vi "Display Telemtery Data.vi"(0 "Instance Details":T1) -> (17 "TX Queue State":i32(slide) scale=0.0..50.0, 18 "Initialisation Progress":u8(slide) scale=0.0..100.0, 19 "RX Queue State":i32(slide) scale=0.0..50.0, 20 "Drone Information Out":T4={"Heart Beat"=FALSE, "Aircraft ID"=0, "Tag ID"="", "System Status"="", "Base Mode"={"Custom Mode"=FALSE, "Test Enabled"=FALSE, "Autonomous Mode"=FALSE, "Guided Mode"=FALSE, "Stabilization Enabled"=FALSE, "HIL Enabled"=FALSE, "Manual Mode"=FALSE, "Arm"=FALSE}, "Armed/Disarmed"=FALSE, "Battery Voltage"=0.0, "Control Mode"=enum."Stabalise", "Initialisation"=0, "Heart Beat Status"=FALSE, "Mode"="", "Mission Uploaded"=FALSE} {"Initialisation" scale=0.0..100.0}, 21 "System Status Out":T9 {"Communication Drop Rate (%)" scale=0.0..100.0; "Battery Remaining (%)" scale=0.0..100.0; "CPU Load (%)" scale=0.0..100.0}, 22 "Status text":string, 23 "Armed/Disarmed":bool, 24 "Aircraft RC Data Out":T8, 25 "Aircraft Att Data Out":T7, 26 "Control Mode":T6=enum."Stabalise")   [LabVIEW 2014]
uses:
  Aircraft Information/Controls/Aircraft Sensor Status Data.ctl
  GUI Design/Indicators/Sensor Status LED CLuster.ctl
  GUI Design/Indicators/Status LED.ctl
  Aircraft Information/Controls/Aircraft Mode.ctl
  Aircraft Information/Controls/Aircraft RC Data.ctl
  Aircraft Information/Controls/Aircraft Attitude Data.ctl
  Aircraft Information/Controls/Drone Information.ctl
  Aircraft Information/Controls/Base Mode.ctl
  Ground Station to Aircraft Coms/SubVI/Aircraft Data Router/Controls/Known Aircraft.ctl
  Ground Station to Aircraft Coms/SubVI/Hardware Driver/Controls/Coms Driver Interface.ctl
  Controls/Telemetry Connection Type.ctl
  Aircraft Information/Sub VI/Get Aircraft Attitude.vi
  Aircraft Information/Sub VI/Get Aircraft RC.vi
  Aircraft Information/Sub VI/Get Aircraft System Status.vi
  Aircraft Information/Sub VI/Get Aircraft Information.vi
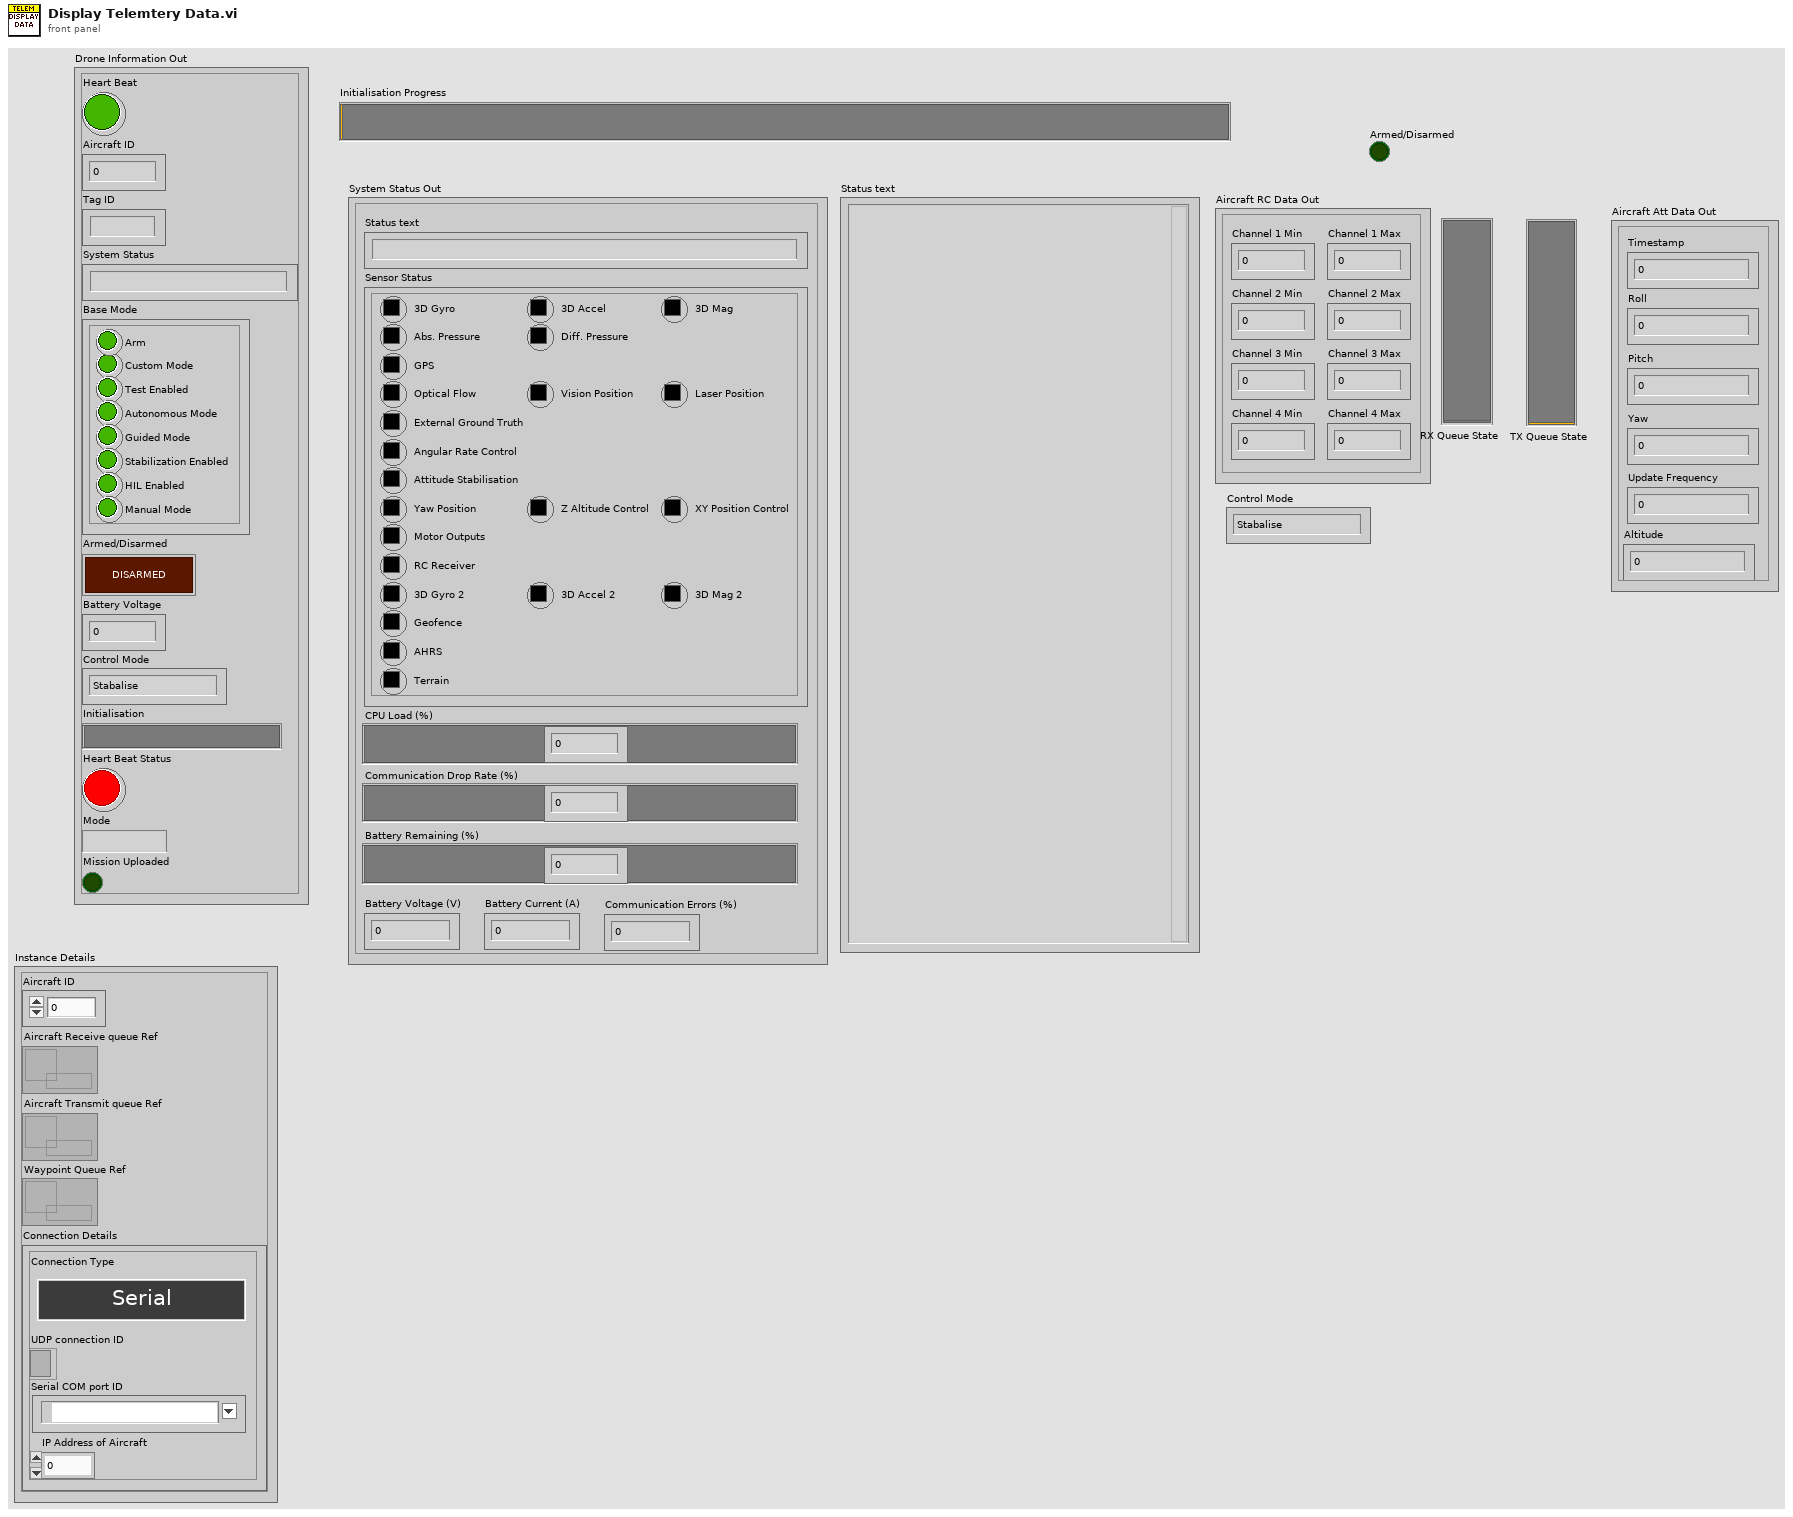
[diagram p1: front panel]
types:
  T1 = typedef "Known Aircraft.ctl" = cluster{"Aircraft ID":u8, "Aircraft Receive queue Ref":refnum<queue>, "Aircraft Transmit queue Ref":refnum<queue>, "Waypoint Queue Ref":refnum<queue>, "Connection Details":T2}
  T2 = typedef "Coms Driver Interface.ctl" = cluster{"Connection Type":T3, "UDP connection ID":refnum<k16>, "Serial COM port ID":refnum<visa-resource-name>, "IP Address of Aircraft":u32}
  T3 = typedef "Telemetry Connection Type.ctl" = enum16{"Serial", "UDP", "TCP"}
  T4 = typedef "Drone Information.ctl" = cluster{"Heart Beat":bool, "Aircraft ID":u8, "Tag ID":string, "System Status":string, "Base Mode":T5, "Armed/Disarmed":bool, "Battery Voltage":dbl, "Control Mode":T6, "Initialisation":u8, "Heart Beat Status":bool, "Mode":string, "Mission Uploaded":bool}
  T5 = typedef "Base Mode.ctl" = cluster{"Custom Mode":bool, "Test Enabled":bool, "Autonomous Mode":bool, "Guided Mode":bool, "Stabilization Enabled":bool, "HIL Enabled":bool, "Manual Mode":bool, "Arm":bool}
  T6 = typedef "Aircraft Mode.ctl" = enum16{"Loiter", "Stabalise", "Failsafe", "Emergency Stop"}
  T7 = typedef "Aircraft Attitude Data.ctl" = cluster{"Roll":sgl, "Pitch":sgl, "Yaw":sgl, "Timestamp":u32, "Update Frequency":dbl, "Altitude":sgl}
  T8 = typedef "Aircraft RC Data.ctl" = cluster{"Channel 1 Min":i16, "Channel 1 Max":i16, "Channel 2 Min":i16, "Channel 2 Max":i16, "Channel 3 Min":i16, "Channel 3 Max":i16, "Channel 4 Min":i16, "Channel 4 Max":i16}
  T9 = typedef "Aircraft Sensor Status Data.ctl" = cluster{"Sensor Status":T10, "CPU Load (%)":dbl, "Battery Voltage (V)":dbl, "Battery Current (A)":dbl, "Battery Remaining (%)":dbl, "Communication Drop Rate (%)":dbl, "Communication Errors (%)":dbl, "Status text":string}
  T10 = typedef "Sensor Status LED CLuster.ctl" = cluster{"3D Gyro":u32, "3D Accel":u32, "3D Mag":u32, "Abs. Pressure":u32, "Diff. Pressure":u32, "GPS":T11, "Optical Flow":u32, "Vision Position":u32, "Laser Position":u32, "External Ground Truth":u32, "Angular Rate Control":u32, "Attitude Stabilisation":u32, "Yaw Position":u32, "Z Altitude Control":u32, "XY Position Control":u32, "Motor Outputs":u32, "RC Receiver":u32, "3D Gyro 2":u32, "3D Accel 2":u32, "3D Mag 2":u32, "Geofence":u32, "AHRS":u32, "Terrain":u32}
  T11 = typedef "Status LED.ctl" = u32
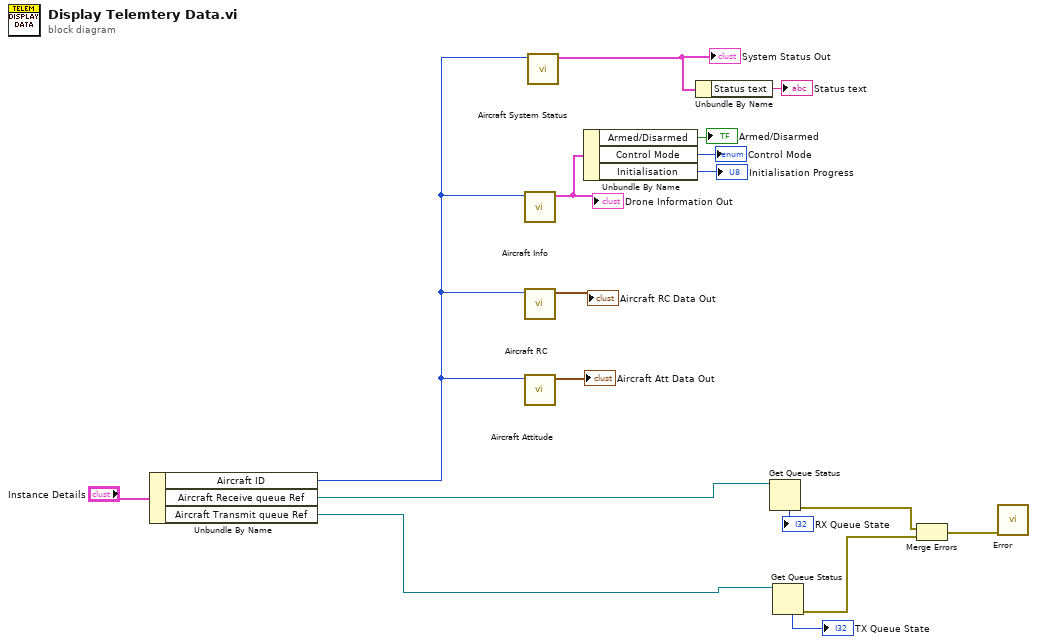
[diagram p0: block diagram]
diagram:
  n1 = Unbundle By Name("Instance Details") -> ("Aircraft ID"=w3:u8, "Aircraft Receive queue Ref"=w2:refnum<queue>, "Aircraft Transmit queue Ref"=w1:refnum<queue>)
  n2 = call-poly "Aircraft Info.vi"("Aircraft ID"=w3) -> ("Aircraft Information Out"=w8:T4)  [unwired: 9 in, 1 out]
  "Drone Information Out" <- w8
  n3 = call-poly "Aircraft RC.vi"("Aircraft ID"=w3) -> ("Aircraft RC Data"=→"Aircraft RC Data Out":T8)  [unwired: 9 in, 1 out]
  n4 = call-poly "Aircraft Attitude.vi"("Aircraft ID"=w3) -> ("Aircraft Att Data Out"=→"Aircraft Att Data Out":T7)  [unwired: 9 in, 1 out]
  n5 = call-poly "Aircraft System Status.vi"("Aircraft ID"=w3) -> ("System Status Out"=w6:T9)  [unwired: 9 in, 1 out]
  "System Status Out" <- w6
  n6 = Unbundle By Name(w8) -> ("Armed/Disarmed"=→"Armed/Disarmed":bool, "Control Mode"=→"Control Mode":T6, "Initialisation"=→"Initialisation Progress":u8)
  n7 = Unbundle By Name(w6) -> ("Status text"=→"Status text":string)
  n8 = Get Queue Status(queue=w2) -> (error out=w13:errorcluster, # elements in queue=→"RX Queue State":i32)  [unwired: 2 in, 6 out]
  n9 = Get Queue Status(queue=w1) -> (error out=w12:errorcluster, # elements in queue=→"TX Queue State":i32)  [unwired: 2 in, 6 out]
  n10 = Merge Errors(w13, w12) -> (w11:errorcluster)
  n11 = call "Error.vi"("Error In"=w11) -> ()  [unwired: 10 in, 1 out]
